vi "GOOP_DrawWirePreview_DrawWire.vi"(7 "WireConfiguration":T1, 10 "Array":cluster{"x":i16, "y":i16}[](array[cluster]), 11 "PictureIn":picture) -> (3 "PictureOut":picture)   [LabVIEW 2020]
uses:
  <resource>/Framework/Providers/Open_GDS/SubVIs/GOOP_WireConfigurationType.ctl
  <resource>/Framework/Providers/Open_GDS/SubVIs/GOOP_WirePattern.ctl
  <vilib>/picture/picture.llb/Draw True-Color Pixmap.vi
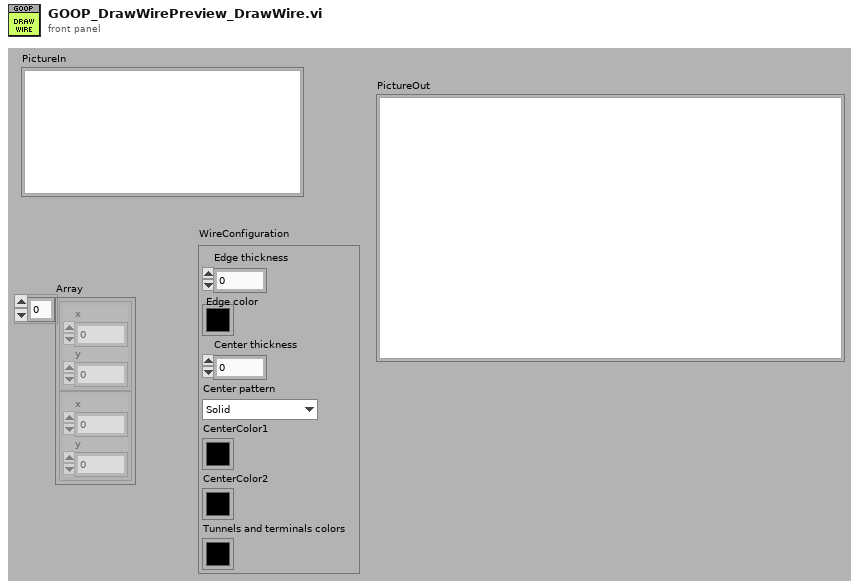
[diagram p1: front panel]
types:
  T1 = typedef "GOOP_WireConfigurationType.ctl" = cluster{"Edge thickness":i32, "Edge color":u32, "Center thickness":i32, "Center pattern":T2, "CenterColor1":u32, "CenterColor2":u32, "Tunnels and terminals colors":u32}
  T2 = typedef "GOOP_WirePattern.ctl" = enum16{"Solid", "Large dash", "Small dash"}
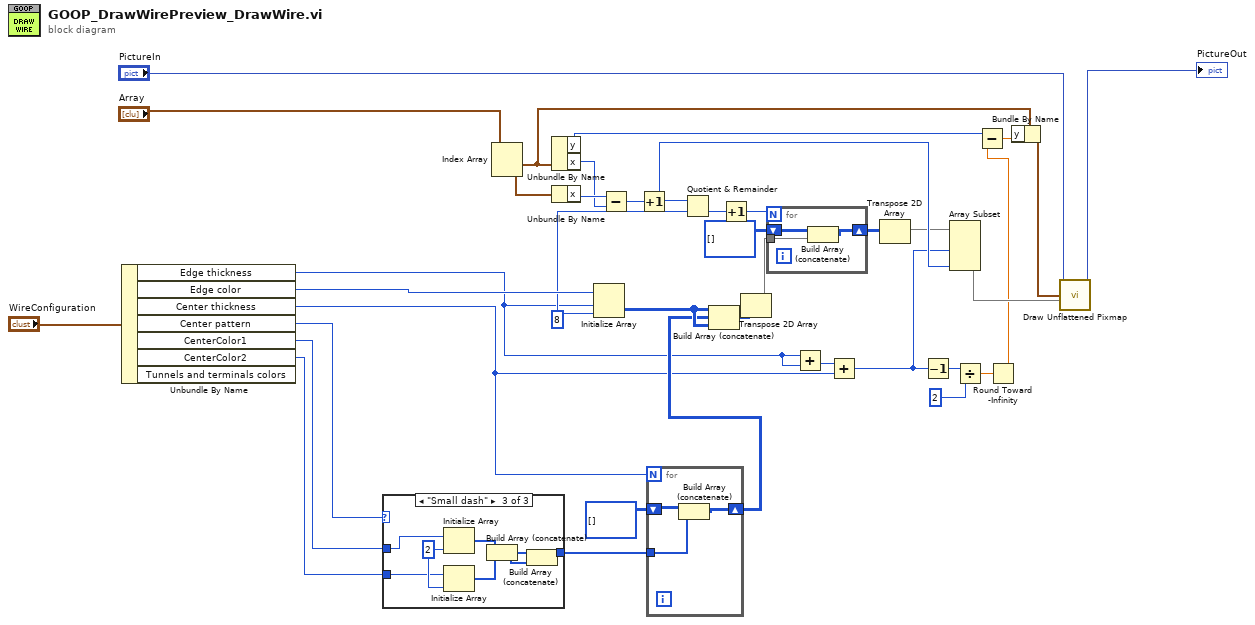
[diagram p0: block diagram]
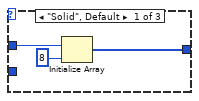
[diagram p2: hidden frame]
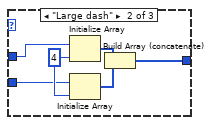
[diagram p3: hidden frame]
diagram:
  w31 = 8 ("dimension size")
  n1 = Unbundle By Name("WireConfiguration") -> ("Edge thickness"=w14:i32, "Edge color"=w32:u32, "Center thickness"=w12:i32, "Center pattern"=w28:T2, "CenterColor1"=w27:u32, "CenterColor2"=w24:u32)  [unwired: 1 out]
  n2 = case shown="\"Small dash\"" w28 {
    tunnel: w27 -> [w40 w46 w53]
    tunnel: [w39 w42 w48] -> w26
    tunnel: w24 -> [_ w45 w52]
    frame "Solid", Default {
      n3 = Initialize Array(w40, 8 ("dimension size")) -> (w39:u32[])
    }
    frame "Large dash" {
      w47 = 4 ("dimension size")
      n4 = Initialize Array(w46, w47) -> (w44:u32[])
      n5 = Initialize Array(w45, w47) -> (w43:u32[])
      n6 = Build Array (concatenate)(w44, w43) -> (w42:u32[])
    }
    frame "Small dash" {
      w54 = 2 ("dimension size")
      n7 = Initialize Array(w53, w54) -> (w51:u32[])
      n8 = Initialize Array(w52, w54) -> (w50:u32[])
      n9 = Build Array (concatenate)(w51, w50) -> (w49:u32[])
      n10 = Build Array (concatenate)(w49, w49) -> (w48:u32[])
    }
  }
  n11 = Index Array(array="Array") -> (element #1=w10:cluster{"x":i16, "y":i16}, element #2=w36:cluster{"x":i16, "y":i16})  [unwired: 2 in]
  n12 = Unbundle By Name(w10) -> ("y"=w11:i16, "x"=w34:i16)
  n13 = Unbundle By Name(w36) -> ("x"=w35:i16)
  n14 = Initialize Array(w32, w14, w31) -> (w30:u32[][])
  n15 = Subtract(x=w35, y=w34) -> (x-y=w33:i16)
  n16 = Increment(x=w33) -> (x+1=w17:i16)
  n17 = for {
    N: w12 -> [_]
    shift-right: [w56] -> w25
    shift-left: u32[][] [] ("initialized array") -> [w57]
    tunnel: w26 -> [w55]
    n18 = Build Array (concatenate)(w57, w55) -> (w56:u32[][])
  }
  n19 = Quotient & Remainder(x=w17, y=w31) -> (floor(x/y)=w23:i32)  [unwired: 1 out]
  n20 = Build Array (concatenate)(w30, w25, w30) -> (w20:u32[][])
  n21 = Increment(x=w23) -> (x+1=w22:i32)
  n22 = Transpose 2D Array(2D array=w20) -> (transposed array=w18:u32[][])
  n23 = for {
    N: w22 -> [_]
    shift-right: [w58] -> w19
    shift-left: u32[][] [] ("initialized array") -> [w60]
    tunnel: w18 -> [w59]
    n24 = Build Array (concatenate)(w60, w59) -> (w58:u32[][])
  }
  n25 = Add(x=w14, y=w14) -> (x+y=w13:i32)
  n26 = Add(x=w13, y=w12) -> (x+y=w7:i32)
  n27 = Transpose 2D Array(2D array=w19) -> (transposed array=w16:u32[][])
  n28 = Decrement(x=w7) -> (x-1=w6:i32)
  n29 = Array Subset(array=w16, length (row)=w7, length (col)=w17) -> (w15:u32[][])  [unwired: 2 in]
  n30 = Divide(x=w6, y=2) -> (x/y=w4:dbl)
  n31 = Round Toward -Infinity(1:w4) -> (0:w3:dbl)
  n32 = Subtract(x=w11, y=w3) -> (x-y=w9:dbl)
  n33 = Bundle By Name(cluster=w10, "y"=w9) -> (w8:cluster{"x":i16, "y":i16})
  n34 = call-poly <vilib>:"Draw Unflattened Pixmap.vi"("picture"="PictureIn", "top left point(0, 0)"=w8, "data (RGB format)"=w15) -> ("new picture"=→"PictureOut":picture)  [unwired: 6 in]
